vi "datasets.list.vi"(8 "error in":errorcluster, 11 "asset in":refnum<class "asset.lvclass">) -> (0 "error out":errorcluster, 2 "datasets":map{string, refnum<class "dataset.lvclass">}(c390), 3 "asset out":refnum<class "asset.lvclass">)   [LabVIEW 2020, in "asset.lvclass"]
uses:
  asset.lvclass
  asset.lvclass/asset.ctl
  datascopes.get.vi
  Nominal Client/datasources/dataset/dataset.lvclass
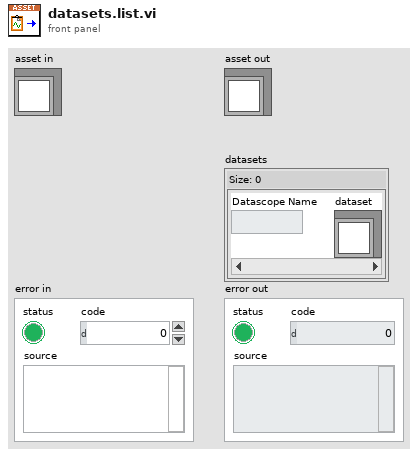
[diagram p1: front panel]
types:
  T1 = typedef "dataScopes.lvlib/data_scopes.ctl" = T2[]
  T2 = typedef "dataScopes.lvlib/data_scope.ctl" = cluster{"dataScopeName":string, "dataSource":T3, "seriesTags":map{string, string}, "offset":T5}
  T3 = typedef "dataScopes.lvlib/data_source.ctl" = cluster{"type":T4, "rid":string}
  T4 = typedef "dataScopes.lvlib/type.ctl" = enum16{"dataset", "connection", "logSet", "video"}
  T5 = typedef "dataScopes.lvlib/offset.ctl" = cluster{"seconds":i32, "nanos":i32, "picos":i32}
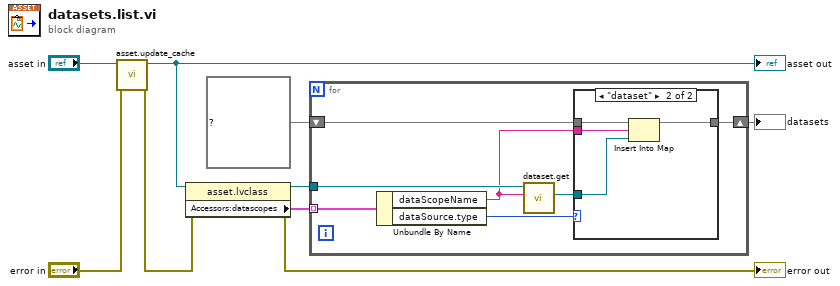
[diagram p0: block diagram]
diagram:
  n1 = call "asset.update_cache.vi"("error in"="error in", "asset in"="asset in") -> ("error out"=w5:errorcluster, "asset out"=w4:refnum<class "asset.lvclass">)  [unwired: 8 in]
  "asset out" <- w4
  n2 = property class="asset.lvclass"(reference=w4, error in=w5) -> (reference out=w3:refnum<class "asset.lvclass">, error out=→"error out":errorcluster, "Accessors:datascopes"=w9:T1)
  n3 = for {
    tunnel: w9 -> [w16] mode=indexing
    tunnel: w3 -> [w15]
    shift-right: [w12] -> w1
    shift-left: map{string, refnum<class "dataset.lvclass">} {} ("map in") -> [w13]
    n4 = Unbundle By Name(w16) -> ("dataScopeName"=w11:string, "dataSource.type"=w14:T4)
    n5 = call "dataset.get.vi"("Datascope Name"=w11, "asset in"=w15) -> ("dataset"=w10:refnum<class "dataset.lvclass">)  [unwired: 7 in, 2 out]
    n6 = case shown="\"dataset\"" w14 {
      tunnel: w13 -> [w17 w21]
      tunnel: [w17 w20] -> w12
      tunnel: w11 -> [_ w19]
      tunnel: w10 -> [_ w18]
      frame Default {
      }
      frame "dataset" {
        n7 = Insert Into Map(map in=w21, key=w19, value=w18) -> (map out=w20:map{string, refnum<class "dataset.lvclass">})  [unwired: 2 out]
      }
    }
  }
  "datasets" <- w1
